vi "Format Text.vi"(7 "Debug Level":T1=enum."INFO", 8 "error in (no error)":errorcluster, 10 "Log Text":string, 11 "Logger in":refnum<class "Logger.lvclass">) -> (0 "error out":errorcluster, 1 "Log Output":string, 3 "Logger out":refnum<class "Logger.lvclass">)   [LabVIEW 2025, in "LV Logging.lvlib" / "Logger.lvclass"]
uses:
  Logger.lvclass
  Type Defs/Debug Level.ctl
  Logger.lvclass/Logger.ctl
  LV Logging.lvlib
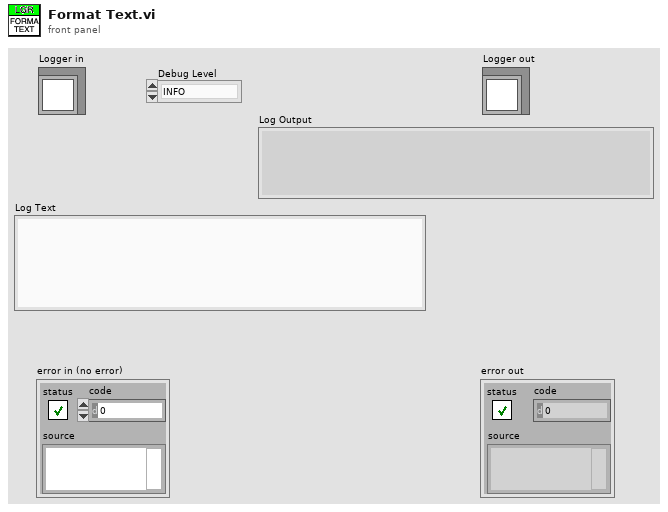
[diagram p1: front panel]
types:
  T1 = typedef "LV Logging.lvlib/Debug Level.ctl" = enum16{"DEBUG", "INFO", "WARN", "ERROR", "FATAL"}
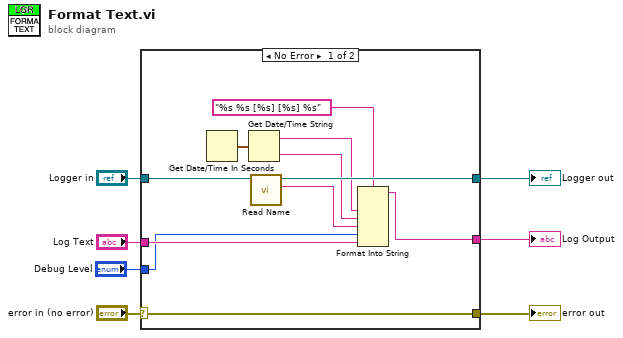
[diagram p0: block diagram]
diagram:
  n1 = case shown="No Error" "error in (no error)" {
    selector: "error in (no error)" -> [w18 w20]
    tunnel: [w18 w20] -> w5
    tunnel: [w16 w19] -> w4
    tunnel: "Logger in" -> [w17 w19]
    tunnel: "Log Text" -> [w14 _]
    tunnel: [w9 _] -> w2
    tunnel: "Debug Level" -> [w8 _]
    frame No Error {
      n2 = Get Date/Time In Seconds() -> (seconds since 1Jan1904=w12:timestamp)
      n3 = Get Date/Time String(seconds (now)=w12) -> (date string=w10:string, time string=w11:string)  [unwired: 2 in]
      n4 = call "Read Name.vi"("Logger in"=w17) -> ("Name"=w15:string, "Logger out"=w16:refnum<class "Logger.lvclass">)  [unwired: 8 in, 1 out]
      n5 = Format Into String(format string="%s %s [%s] [%s] %s", w10, w11, w15, w8, w14) -> (resulting string=w9:string)  [unwired: 2 in, 1 out]
    }
    frame Error {
    }
  }
  "error out" <- w5
  "Logger out" <- w4
  "Log Output" <- w2
